vi "trash_Connect.vi"(8 "error in (no error)":errorcluster, 10 "Connection Name":string, 11 "RTFIFOChannel in":refnum<class "RTFIFOChannel.lvclass">) -> (0 "error out":errorcluster, 3 "RTFIFOChannel out":refnum<class "RTFIFOChannel.lvclass">)   [LabVIEW 2021]
uses:
  RTFIFOChannel.lvclass
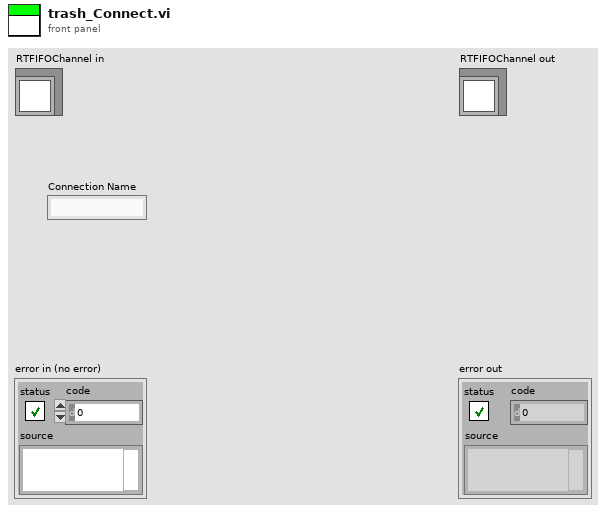
[diagram p1: front panel]
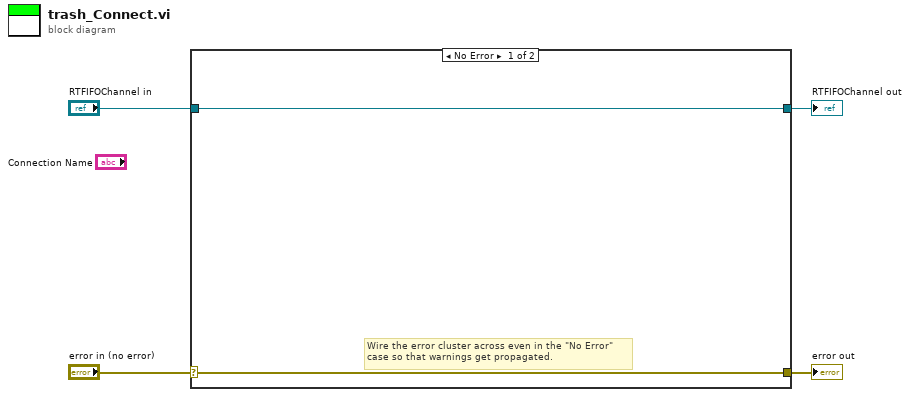
[diagram p0: block diagram]
diagram:
  n1 = case shown="No Error" "error in (no error)" {
    selector: "error in (no error)" -> [w5 w8]
    tunnel: [w5 w8] -> w3
    tunnel: [w6 w7] -> w1
    tunnel: "RTFIFOChannel in" -> [w6 w7]
    frame No Error {
      # "Wire the error cluster across even in the \"No Error\"\ncase so that warnings get propagated."
    }
    frame Error {
    }
  }
  "error out" <- w3
  "RTFIFOChannel out" <- w1
